vi "Read Unit ID.vi"(8 "error in":errorcluster, 11 "transmission data unit in":refnum<class "Transmission Data Unit.lvclass">) -> (0 "error out":errorcluster, 2 "unit ID":u8, 3 "transmission data unit out":refnum<class "Transmission Data Unit.lvclass">)   [LabVIEW 2013, in "Modbus Library - Advance.lvlib" / "Transmission Data Unit.lvclass"]
doc: "Accessor VI for unit ID."
uses:
  Transmission Data Unit.lvclass
  Transmission Data Unit.lvclass/Transmission Data Unit.ctl
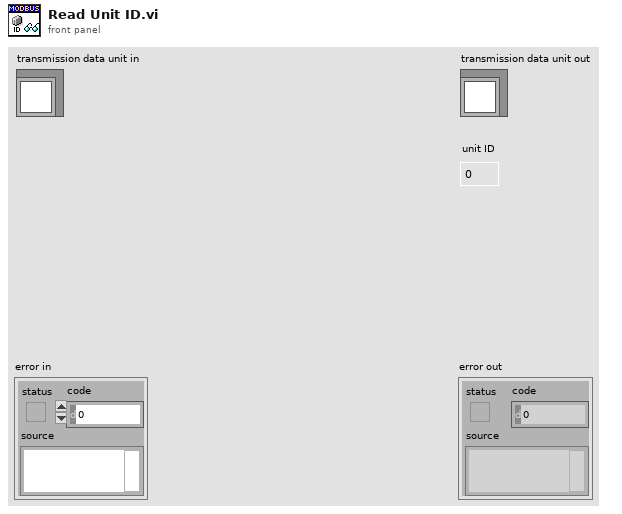
[diagram p1: front panel]
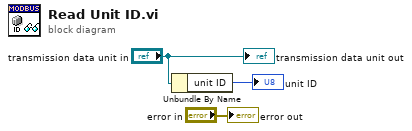
[diagram p0: block diagram]
diagram:
  n1 = Unbundle By Name("transmission data unit in") -> ("unit ID"=→"unit ID":u8)
  "error out" <- "error in"
  "transmission data unit out" <- "transmission data unit in"
